vi "Car Wash.vi"() -> ()   [LabVIEW 2021]
doc: "Use this template to build a queued message handler design pattern."
uses:
  Wash-types.ctl
  Classes/Attributes.lvclass
panel:
  out "Ind.":T1
  in  "Move to Air Dry":bool
  in  "Move to Main Wash":bool
  in  "Underbody Wash":bool
  in  "Stop":bool
  in  "Economy":bool
  in  "Deluxe":bool
  in  "error in":errorcluster
  out "error out":errorcluster
  # "MASTER MONITORING"
  # "Sequence Indicators"
  # "MASTER CONTROLS"
  # "Purchase Selection"
  # "Positioning Switches"
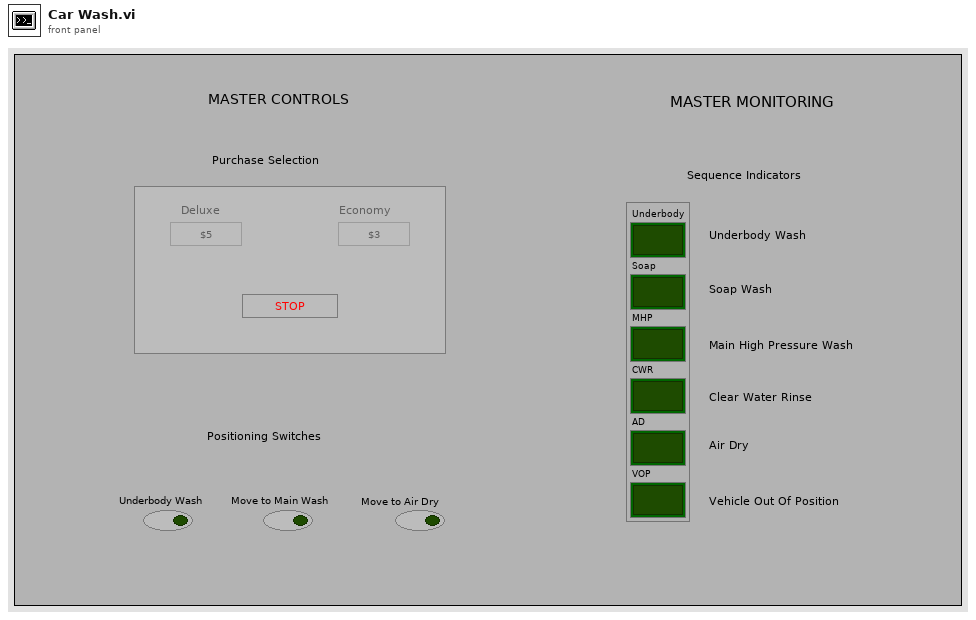
[diagram p1: front panel]
types:
  T1 = typedef "Wash-types.ctl" = cluster{"Underbody":bool, "Soap":bool, "MHP":bool, "CWR":bool, "AD":bool, "VOP":bool}
  T2 = cluster{"UB":bool, "Soap":bool, "MHP":bool, "CWR":bool, "AD":bool, "VOP":bool}
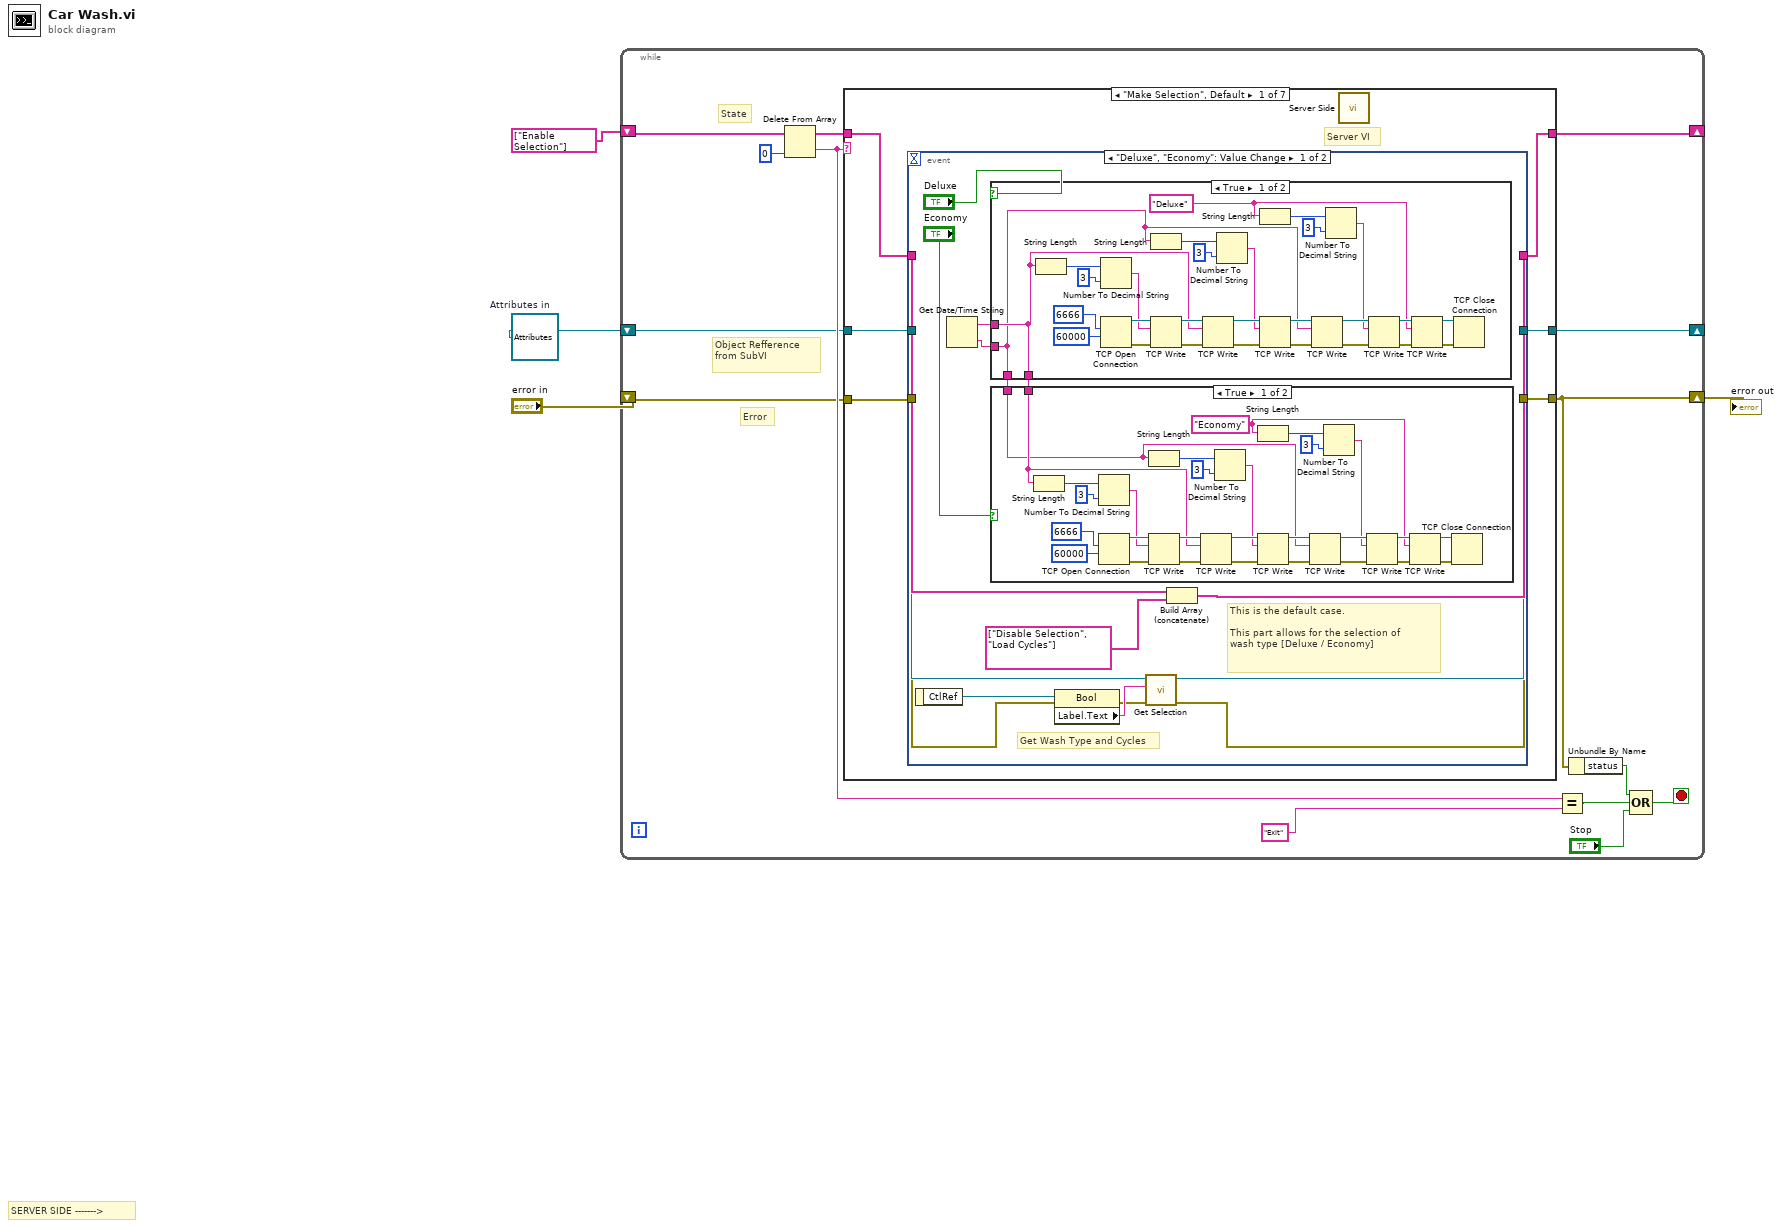
[diagram p0: block diagram]
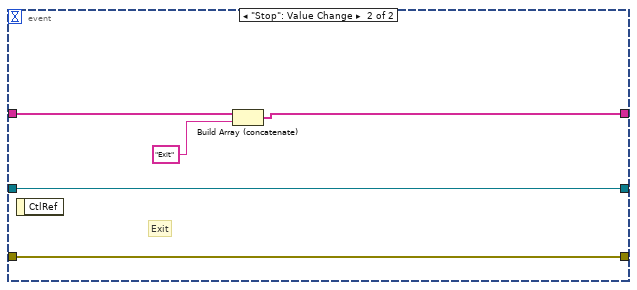
[diagram p4: hidden frame]
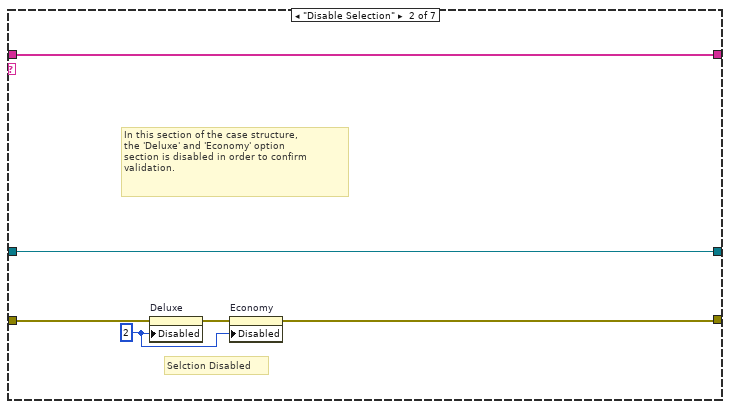
[diagram p5: hidden frame]
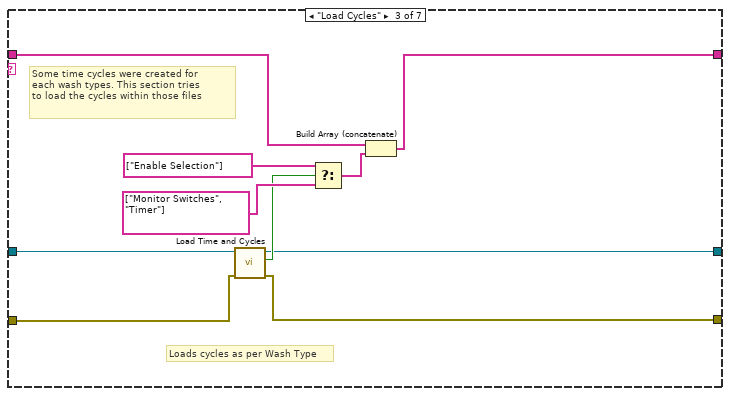
[diagram p6: hidden frame]
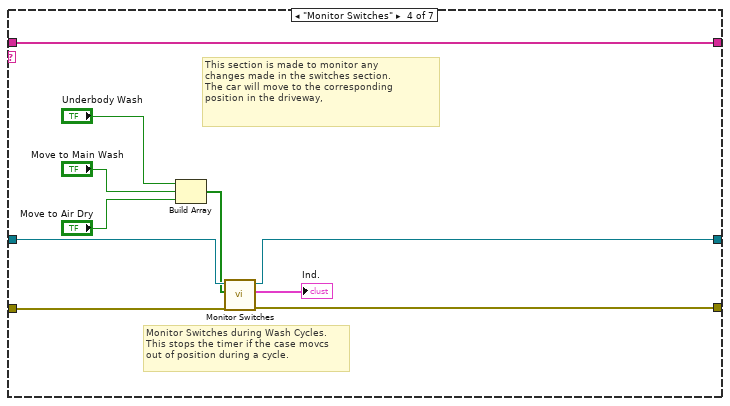
[diagram p7: hidden frame]
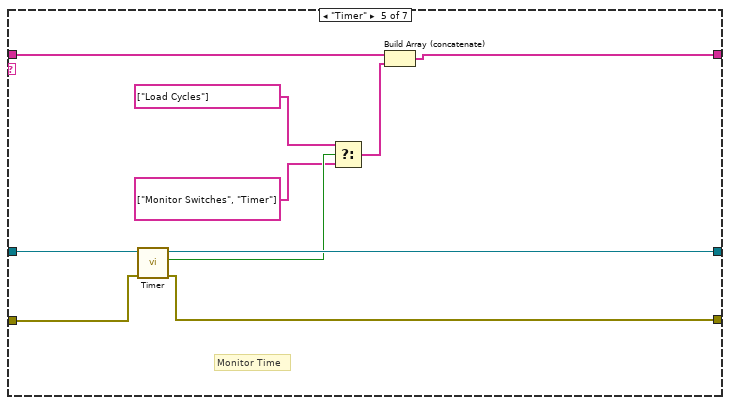
[diagram p8: hidden frame]
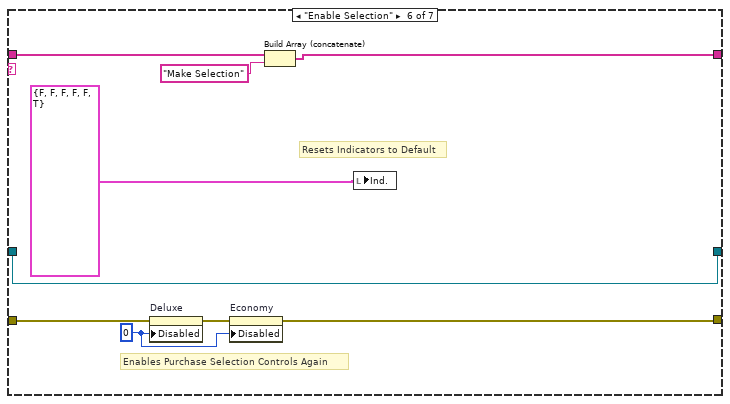
[diagram p9: hidden frame]
diagram:
  w3 = refnum<class "Attributes.lvclass"> refnum  # Attributes in
  # "SERVER SIDE ------->"
  n1 = while {
    shift-right: [w15] -> _
    shift-left: string[] ["Enable Selection"] -> [w18]
    shift-right: [w11] -> _
    shift-left: w3 -> [w12]
    shift-right: [w7] -> w1
    shift-left: "error in" -> [w10]
    stop <- w5 stop-if-true
    # "State"
    # "Error"
    # "Object Refference\nfrom SubVI"
    n2 = Delete From Array(array=w18, index=0) -> (deleted portion=w17:string, array with subset deleted=w16:string[])  [unwired: 1 in]
    n3 = case shown="\"Make Selection\", Default" w17 {
      tunnel: w16 -> [w24 w104 w119 w124 w139 w143 w151]
      tunnel: [w23 w104 w118 w124 w138 w142 w151] -> w15
      tunnel: w12 -> [w22 w105 w117 w129 w136 w144 w150]
      tunnel: [w21 w105 w111 w126 w135 w144 w150] -> w11
      tunnel: w10 -> [w20 w108 w116 w128 w134 w147 w149]
      tunnel: [w19 w107 w110 w127 w133 w146 w149] -> w7
      frame "Make Selection", Default {
        # "Server VI"
        n4 = event shown="[0] \"Deluxe\", \"Economy\": Value Change" {
          selector: _ -> [_ _]
          dyn-events: _ -> [_ _]
          timeout: _ -> [_ _]
          tunnel: w24 -> [w40 w100]
          tunnel: [w39 w99] -> w23
          tunnel: w22 -> [w36 w103]
          tunnel: [w34 w103] -> w21
          tunnel: w20 -> [w33 w102]
          tunnel: [w32 w102] -> w19
          event "Deluxe", "Economy": Value Change {
            # "This is the default case.\n\nThis part allows for the selection of \nwash type [Deluxe / Economy]"
            # "Get Wash Type and Cycles"
            n5 = event-data() -> ("CtlRef"=w38:refnum<vi>)  [unwired: 1 in]
            n6 = Get Date/Time String() -> (date string=w28:string, time string=w26:string)  [unwired: 3 in]
            n7 = case shown="True" "Deluxe" {
              tunnel: w28 -> [w70 w97]
              tunnel: [w70 w97] -> w27
              tunnel: w26 -> [w69 w98]
              tunnel: [w69 w98] -> w25
              frame True {
                w71 = "Deluxe"
                n8 = String Length(string=w70) -> (length=w90:i32)
                n9 = Number To Decimal String(number=w90, width (-)=i16 3) -> (decimal integer string=w88:string)
                n10 = TCP Open Connection(remote port or service name=u16 6666, timeout ms (60000)=60000) -> (connection ID=w92:refnum<k5>, error out=w94:errorcluster)  [unwired: 3 in]
                n11 = String Length(string=w69) -> (length=w76:i32)
                n12 = TCP Write(connection ID=w92, data in=w88, error in (no error)=w94) -> (connection ID out=w91:refnum<k5>, error out=w93:errorcluster)  [unwired: 1 in, 1 out]
                n13 = TCP Write(connection ID=w91, data in=w70, error in (no error)=w93) -> (connection ID out=w82:refnum<k5>, error out=w85:errorcluster)  [unwired: 1 in, 1 out]
                n14 = Number To Decimal String(number=w76, width (-)=i16 3) -> (decimal integer string=w73:string)
                n15 = String Length(string=w71) -> (length=w75:i32)
                n16 = TCP Write(connection ID=w82, data in=w73, error in (no error)=w85) -> (connection ID out=w81:refnum<k5>, error out=w87:errorcluster)  [unwired: 1 in, 1 out]
                n17 = TCP Write(connection ID=w81, data in=w69, error in (no error)=w87) -> (connection ID out=w80:refnum<k5>, error out=w84:errorcluster)  [unwired: 1 in, 1 out]
                n18 = Number To Decimal String(number=w75, width (-)=i16 3) -> (decimal integer string=w72:string)
                n19 = TCP Write(connection ID=w80, data in=w72, error in (no error)=w84) -> (connection ID out=w79:refnum<k5>, error out=w86:errorcluster)  [unwired: 1 in, 1 out]
                n20 = TCP Write(connection ID=w79, data in=w71, error in (no error)=w86) -> (connection ID out=w78:refnum<k5>, error out=w83:errorcluster)  [unwired: 1 in, 1 out]
                n21 = TCP Close Connection(connection ID=w78, error in (no error)=w83) -> ()  [unwired: 1 in, 2 out]
              }
              frame False {
              }
            }
            n22 = case shown="True" "Economy" {
              tunnel: w27 -> [w42 _]
              tunnel: w25 -> [w41 _]
              frame True {
                w43 = "Economy"
                n23 = String Length(string=w42) -> (length=w62:i32)
                n24 = Number To Decimal String(number=w62, width (-)=i16 3) -> (decimal integer string=w60:string)
                n25 = TCP Open Connection(remote port or service name=u16 6666, timeout ms (60000)=60000) -> (connection ID=w64:refnum<k5>, error out=w66:errorcluster)  [unwired: 3 in]
                n26 = String Length(string=w41) -> (length=w48:i32)
                n27 = TCP Write(connection ID=w64, data in=w60, error in (no error)=w66) -> (connection ID out=w63:refnum<k5>, error out=w65:errorcluster)  [unwired: 1 in, 1 out]
                n28 = TCP Write(connection ID=w63, data in=w42, error in (no error)=w65) -> (connection ID out=w54:refnum<k5>, error out=w57:errorcluster)  [unwired: 1 in, 1 out]
                n29 = Number To Decimal String(number=w48, width (-)=i16 3) -> (decimal integer string=w45:string)
                n30 = String Length(string=w43) -> (length=w47:i32)
                n31 = TCP Write(connection ID=w54, data in=w45, error in (no error)=w57) -> (connection ID out=w53:refnum<k5>, error out=w59:errorcluster)  [unwired: 1 in, 1 out]
                n32 = TCP Write(connection ID=w53, data in=w41, error in (no error)=w59) -> (connection ID out=w52:refnum<k5>, error out=w56:errorcluster)  [unwired: 1 in, 1 out]
                n33 = Number To Decimal String(number=w47, width (-)=i16 3) -> (decimal integer string=w44:string)
                n34 = TCP Write(connection ID=w52, data in=w44, error in (no error)=w56) -> (connection ID out=w51:refnum<k5>, error out=w58:errorcluster)  [unwired: 1 in, 1 out]
                n35 = TCP Write(connection ID=w51, data in=w43, error in (no error)=w58) -> (connection ID out=w50:refnum<k5>, error out=w55:errorcluster)  [unwired: 1 in, 1 out]
                n36 = TCP Close Connection(connection ID=w50, error in (no error)=w55) -> ()  [unwired: 1 in, 2 out]
              }
              frame False {
              }
            }
            n37 = property class="Bool"(reference=w38, error in=w33) -> (error out=w35:errorcluster, "Label.Text"=w37:string)  [unwired: 1 out]
            n38 = call-dynamic "Get Selection.vi"("error in (no error)"=w35, "Wash"=w37, "Attributes in"=w36) -> ("error out"=w32:errorcluster, "Attributes out"=w34:refnum<class "Attributes.lvclass">)  [unwired: 7 in]
            n39 = Build Array (concatenate)(w40, string[] ["Disable Selection", "Load Cycles"]) -> (w39:string[])
          }
          event "Stop": Value Change {
            # "Exit"
            n40 = event-data() -> ()  [unwired: 1 in, 1 out]
            n41 = Build Array (concatenate)(w100, "Exit") -> (w99:string[])
          }
        }
        n42 = call "Server Side.vi"() -> ()  [unwired: 12 in]
      }
      frame "Disable Selection" {
        w106 = u8 2 ("Disabled")
        # "Selction Disabled"
        # "In this section of the case structure,\nthe 'Deluxe' and 'Economy' option\nsection is disabled in order to confirm\nvalidation."
        n43 = property on="Deluxe" class="Bool"(error in=w108, "Disabled"=w106) -> (error out=w109:errorcluster)  [unwired: 1 in, 1 out]
        n44 = property on="Economy" class="Bool"(error in=w109, "Disabled"=w106) -> (error out=w107:errorcluster)  [unwired: 1 in, 1 out]
      }
      frame "Load Cycles" {
        # "Some time cycles were created for\neach wash types. This section tries\nto load the cycles within those files"
        # "Loads cycles as per Wash Type"
        n45 = call-dynamic "Load Time and Cycles.vi"("error in (no error)"=w116, "Attributes in"=w117) -> ("error out"=w110:errorcluster, "Wash Complete"=w112:bool, "Attributes out"=w111:refnum<class "Attributes.lvclass">)  [unwired: 7 in]
        n46 = Select(t=string[] ["Enable Selection"], s=w112, f=string[] ["Monitor Switches", "Timer"]) -> (s? t:f=w115:string[])
        n47 = Build Array (concatenate)(w119, w115) -> (w118:string[])
      }
      frame "Monitor Switches" {
        # "This section is made to monitor any\nchanges made in the switches section.\nThe car will move to the corresponding \nposition in the driveway,"
        # "Monitor Switches during Wash Cycles.\nThis stops the timer if the case movcs\nout of position during a cycle."
        n48 = Build Array("Underbody Wash", "Move to Main Wash", "Move to Air Dry") -> (w125:bool[])
        n49 = call-dynamic "Monitor Switches.vi"("error in (no error)"=w128, "Switches"=w125, "Attributes in"=w129) -> ("error out"=w127:errorcluster, "Indicators"=→"Ind.":T2, "Attributes out"=w126:refnum<class "Attributes.lvclass">)  [unwired: 6 in]
      }
      frame "Timer" {
        # "Monitor Time"
        n50 = call-dynamic "Timer.vi"("error in (no error)"=w134, "Attributes in"=w136) -> ("error out"=w133:errorcluster, "Complete?"=w132:bool, "Attributes out"=w135:refnum<class "Attributes.lvclass">)  [unwired: 7 in]
        n51 = Select(t=string[] ["Load Cycles"], s=w132, f=string[] ["Monitor Switches", "Timer"]) -> (s? t:f=w137:string[])
        n52 = Build Array (concatenate)(w139, w137) -> (w138:string[])
      }
      frame "Enable Selection" {
        w145 = u8 0 ("Disabled")
        # "Resets Indicators to Default"
        # "Enables Purchase Selection Controls Again"
        n53 = property on="Deluxe" class="Bool"(error in=w147, "Disabled"=w145) -> (error out=w148:errorcluster)  [unwired: 1 in, 1 out]
        n54 = property on="Economy" class="Bool"(error in=w148, "Disabled"=w145) -> (error out=w146:errorcluster)  [unwired: 1 in, 1 out]
        n55 = Build Array (concatenate)(w143, "Make Selection") -> (w142:string[])
        n56 = local write "Ind."(T1 {"Underbody"=FALSE, "Soap"=FALSE, "MHP"=FALSE, "CWR"=FALSE, "AD"=FALSE, "VOP"=TRUE} ("Ind.")) -> ()
      }
      frame "Exit" {
        # "There is nothing in this structure. The program will now wait for a prompt\nfrom the 'STOP' button in order to close."
        # "This section closes the program"
      }
    }
    n57 = Equal?(x=w17, y="Exit") -> (x = y?=w9:bool)
    n58 = Unbundle By Name(w7) -> ("status"=w8:bool)
    n59 = Compound Arithmetic op=OR(w8, w9, "Stop") -> (w5:bool)
  }
  "error out" <- w1
